vi "Create Counter Input PWM Module.vi"   [LabVIEW 2020, in "Scan Engine Scripting.lvlib"]
doc: "Creates and configures an instance of a counter input Pulse Width Modulation (PWM) module that can be used to set a slot in a Scan Engine custom device chassis."
uses:
  Scan Engine Scripting.lvlib
  Modules/NI 9423/NI 9423.lvclass
  Modules/NI 9437/NI 9437.lvclass
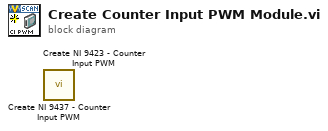
[diagram p0: block diagram]
diagram:
  n1 = call "Create NI 9437 - Counter Input PWM.vi"() -> ()  [unwired: 10 in, 2 out]
  n2 = call "Create NI 9423 - Counter Input PWM.vi"() -> ()  [unwired: 10 in, 2 out]
